vi "SysDef.Globals.vi"() -> ()   [LabVIEW 2015, in "System Definition Utilities.lvlib"]
uses:
  System Definition Utilities.lvlib
panel:
  in  "Version":string="1.0.0"
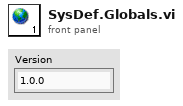
[diagram p1: front panel]
diagram:
